vi "Add Value to Buffer.vi"(8 "error in (no error)":errorcluster, 10 "Encoder Position":dbl, 11 "Linear Encoder in":refnum<class "Linear Encoder.lvclass">) -> (0 "error out":errorcluster, 3 "Linear Encoder out":refnum<class "Linear Encoder.lvclass">)   [LabVIEW 2020, in "Linear Encoder.lvlib" / "Linear Encoder.lvclass"]
uses:
  Linear Encoder.lvclass
  Linear Encoder.lvclass/Linear Encoder.ctl
  <vilib>/ActorFramework/Actor/Actor.lvclass
  C:/Program Files (x86)/National Instruments/LabVIEW 2020/vi.lib/ActorFramework/Actor/Actor.lvclass
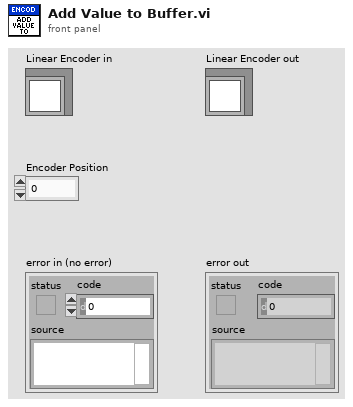
[diagram p1: front panel]
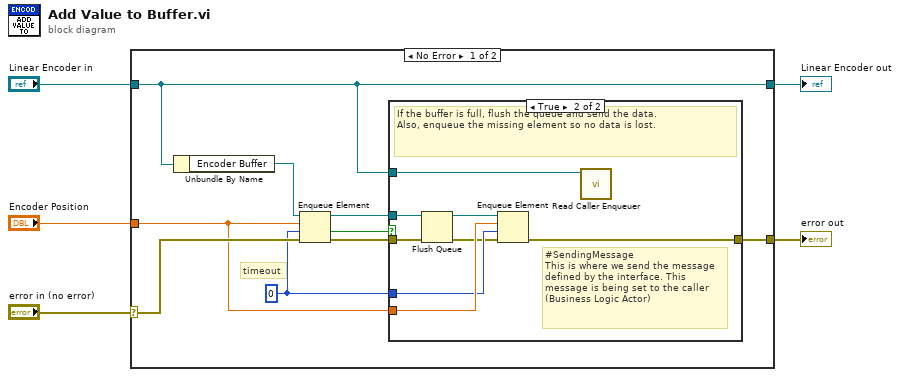
[diagram p0: block diagram]
diagram:
  n1 = case shown="No Error" "error in (no error)" {
    selector: "error in (no error)" -> [w11 w25]
    tunnel: [w7 w25] -> w4
    tunnel: [w6 w24] -> w2
    tunnel: "Linear Encoder in" -> [w6 w24]
    tunnel: "Encoder Position" -> [w9 _]
    frame No Error {
      w8 = 0 ("timeout in ms (-1)")
      # "timeout"
      n2 = Unbundle By Name(w6) -> ("Encoder Buffer"=w14:refnum<queue>)
      n3 = Enqueue Element(queue=w14, element=w9, timeout in ms (-1)=w8, error in (no error)=w11) -> (queue out=w13:refnum<queue>, timed out?=w10:bool, error out=w12:errorcluster)
      n4 = case shown="True" w10 {
        tunnel: w13 -> [_ w23]
        tunnel: w12 -> [w15 w22]
        tunnel: w9 -> [_ w20]
        tunnel: w8 -> [_ w19]
        tunnel: [w15 w16] -> w7
        tunnel: w6 -> [_ w17]
        frame False {
        }
        frame True {
          # "#SendingMessage\nThis is where we send the message defined by the interface. This message is being set to the caller (Business Logic Actor)"
          # "If the buffer is full, flush the queue and send the data.\nAlso, enqueue the missing element so no data is lost."
          n5 = Flush Queue(queue=w23, error in (no error)=w22) -> (queue out=w21:refnum<queue>, error out=w18:errorcluster)  [unwired: 1 out]
          n6 = Enqueue Element(queue=w21, element=w20, timeout in ms (-1)=w19, error in (no error)=w18) -> (error out=w16:errorcluster)  [unwired: 2 out]
          n7 = call <vilib>:"Read Caller Enqueuer.vi"("Actor"=w17) -> ()  [unwired: 10 in, 1 out]
        }
      }
    }
    frame Error {
    }
  }
  "error out" <- w4
  "Linear Encoder out" <- w2
